vi "Open Solver.vi"(8 "error in (no error)":errorcluster, 11 "Solver Path":path) -> (0 "error IO":errorcluster, 3 "Solver VI":T1)   [LabVIEW 2024, in "Wordle Scorer.lvlib"]
uses:
  Wordle Scorer.lvlib
  Solver VI Ref Type.ctl
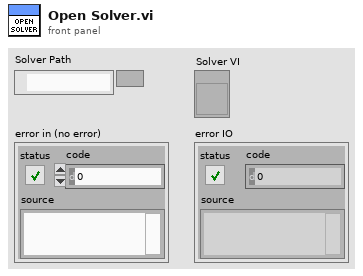
[diagram p1: front panel]
types:
  T1 = typedef "Wordle Scorer.lvlib/Solver VI Ref Type.ctl" = refnum<vi>
  T2 = enum32{"Invalid", "Standard", "Closed", "Hidden", "Minimized", "Maximized"}
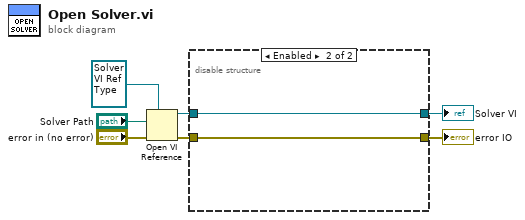
[diagram p0: block diagram]
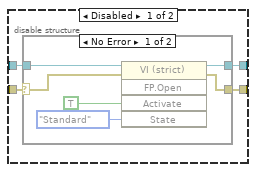
[diagram p2: hidden frame]
diagram:
  n1 = Open VI Reference(type specifier VI Refnum (for type only)=T1 refnum ("Solver VI"), vi path="Solver Path", error in (no error)="error in (no error)") -> (vi reference=w5:T1, error out=w6:errorcluster)  [unwired: 3 in]
  n2 = disable-structure shown="Enabled" {
    disable-tunnel: w6 -> [w11 w20]
    disable-tunnel: w5 -> [w10 w21]
    disable-tunnel: [w9 w20] -> w3
    disable-tunnel: [w8 w21] -> w1
    frame Disabled {
      n3 = case shown="No Error" w11 {
        selector: w11 -> [w13 w19]
        tunnel: w10 -> [w17 w18]
        tunnel: [w12 w19] -> w9
        tunnel: [w14 w18] -> w8
        frame No Error {
          n4 = invoke class="VI (strict)" method="FP.Open"(reference=w17, error in=w13, "Activate"=TRUE ("Activate?"), "State"=T2."Standard") -> (reference out=w14:T1, error out=w12:errorcluster)  [unwired: 1 in, 3 out]
        }
        frame Error {
        }
      }
    }
    frame Enabled {
    }
  }
  "Solver VI" <- w1
  "error IO" <- w3
